vi "FTW-EventLogger-Launch.vi"(0 "LoggerID":string, 5 "Log Directory":path, 7 "Application Name":string, 9 "Disk Thrash Delay (200msec)":u32=200 format="%dmsec", 11 "error in":errorcluster) -> (4 "Event Logger API":refnum<class "FTW-EventLogger-API.lvclass">, 15 "error out":errorcluster)   [LabVIEW 2012, in "FTW-EventLogger-API.lvclass"]
doc: "This method launches a Logger Process which is then referred to based on its LoggerID. Normally in a LabVIEW application, an object's methods would adhere to dataflow with the object wired to the method; however, the Logger Process object likely needs to be accessed by many different portions of your application, and for this reason, it is called by reference, where the LoggerID string refers to the logger.\n\nThis method should be called as one of the very first actions in your application to reasonably ensure the buffer of logged events does not overflow. Events that are logged prior to launching the Logger Process with this method are queued, and will be logged once this process begins."
uses:
  FTW-EventLogger-API.lvclass
  FTW-EventLogger-API.lvclass/FTW-EventLogger-API.ctl
panel:
  # "Inputs"
  # "Outputs"
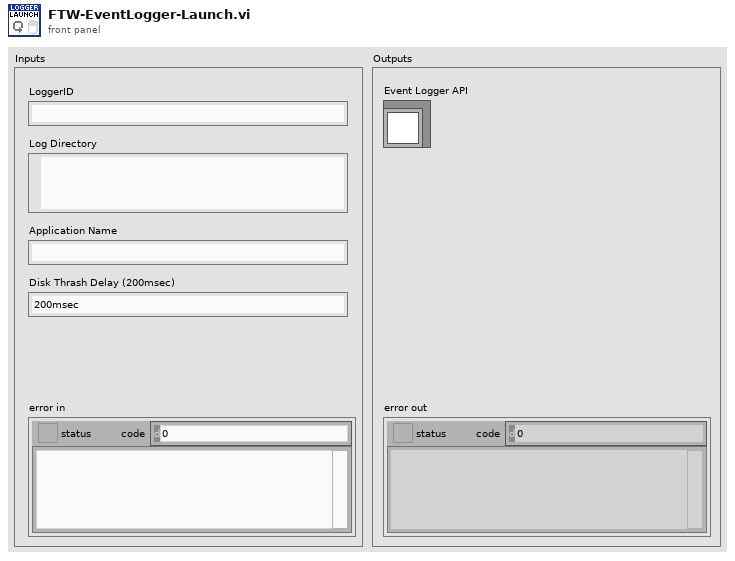
[diagram p1: front panel]
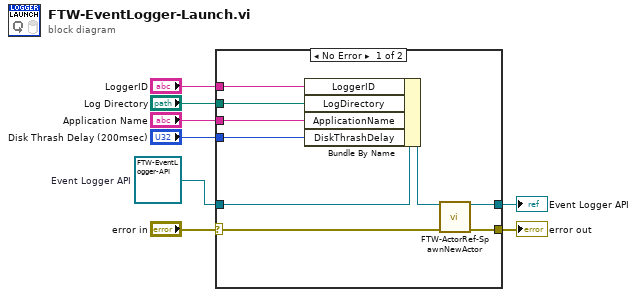
[diagram p0: block diagram]
diagram:
  w1 = refnum<class "FTW-EventLogger-API.lvclass"> refnum  # Event Logger API
  n1 = case shown="No Error" "error in" {
    selector: "error in" -> [w15 w19]
    tunnel: [w14 w19] -> w8
    tunnel: "LoggerID" -> [w11 _]
    tunnel: "Log Directory" -> [w12 _]
    tunnel: "Application Name" -> [w10 _]
    tunnel: "Disk Thrash Delay (200msec)" -> [w9 _]
    tunnel: [w17 w18] -> w2
    tunnel: w1 -> [w16 w18]
    frame No Error {
      n2 = Bundle By Name(cluster=w16, "LoggerID"=w11, "LogDirectory"=w12, "ApplicationName"=w10, "DiskThrashDelay"=w9) -> (w13:refnum<class "FTW-EventLogger-API.lvclass">)
      n3 = call-dynamic "FTW-ActorRef-SpawnNewActor.vi"("Actor Ref Prototype"=w13, "error in"=w15) -> ("Actor Reference"=w17:refnum<class "FTW-EventLogger-API.lvclass">, "error out"=w14:errorcluster)  [unwired: 12 in]
    }
    frame Error {
    }
  }
  "error out" <- w8
  "Event Logger API" <- w2
